vi "check Root Path.vi"(8 "error in (no error)":errorcluster, 11 "Variant Data Manipulation Tests in":refnum<class "Variant Data Manipulation Tests.lvclass">) -> (0 "error out":errorcluster, 3 "Variant Data Manipulation Tests out":refnum<class "Variant Data Manipulation Tests.lvclass">)   [LabVIEW 2017, in "Variant Data Manipulation Tests.lvclass"]
uses:
  Variant Data Manipulation Tests.lvclass
  Source/Path API/Write Value at Path(String).vi
  Source/Path API/Read Value at Path(String).vi
  Source/Path API/Write Label at Path(String).vi
  Source/Variant Data Manipulation.lvlib
  <vilib>/Utility/Data Type/NI_Data Type.lvlib
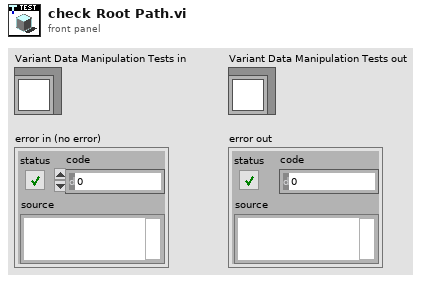
[diagram p1: front panel]
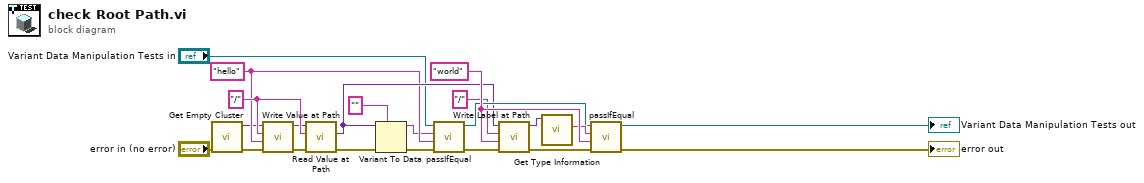
[diagram p0: block diagram]
diagram:
  w20 = "world" ("Name")
  w9 = "hello"
  w11 = "/" ("Path in")
  n1 = call "Get Empty Cluster.vi"("error in (no error)"="error in (no error)") -> ("error out"=w2:errorcluster, "Variant (Cluster) out"=w3:variant)  [unwired: 9 in]
  n2 = call-poly "Write Value at Path.vi"("error in (no error)"=w2, "Element in"=w9, "Path String"=w11, "Variant in"=w3) -> ("error out"=w5:errorcluster, "Variant out"=w4:variant)  [unwired: 6 in]
  n3 = call-poly "Read Value at Path.vi"("error in (no error)"=w5, "Path String"=w11, "Variant in"=w4) -> ("error out"=w6:errorcluster, "Element out"=w13:variant)  [unwired: 6 in, 1 out]
  n4 = Variant To Data(error in=w6, type="" ("Path in"), Variant=w13) -> (data=w8:string, error out=w10:errorcluster)
  n5 = call-dynamic "passIfEqual.vi"("error in (no error)"=w10, "y"=w9, "x"=w8, "TestCase in"="Variant Data Manipulation Tests in") -> ("error out"=w15:errorcluster, "TestCase out"=w16:refnum<class "Variant Data Manipulation Tests.lvclass">)  [unwired: 6 in]
  n6 = call-poly "Write Label at Path.vi"("error in (no error)"=w15, "Name"=w20, "Path String"="/" ("Path in"), "Variant in"=w13) -> ("error out"=w17:errorcluster, "Variant out"=w18:variant)  [unwired: 6 in]
  n7 = call <vilib>:"Get Type Information.vi"("Variant"=w18) -> ("Name"=w19:string)  [unwired: 6 in, 4 out]
  n8 = call-dynamic "passIfEqual.vi"("error in (no error)"=w17, "y"=w20, "x"=w19, "TestCase in"=w16) -> ("error out"=→"error out":errorcluster, "TestCase out"=→"Variant Data Manipulation Tests out":refnum<class "Variant Data Manipulation Tests.lvclass">)  [unwired: 6 in]
